vi "Exit.vi"(8 "error in (no error)":errorcluster, 11 "SV_Publisher in":refnum<class "SV_Publisher.lvclass">) -> (0 "error out":errorcluster, 3 "SV_Publisher out":refnum<class "SV_Publisher.lvclass">)   [LabVIEW 2019, in "SV_Publisher.lvclass"]
uses:
  SV_Publisher.lvclass
  Data.ctl
  SV_Publisher.lvclass/SV_Publisher.ctl
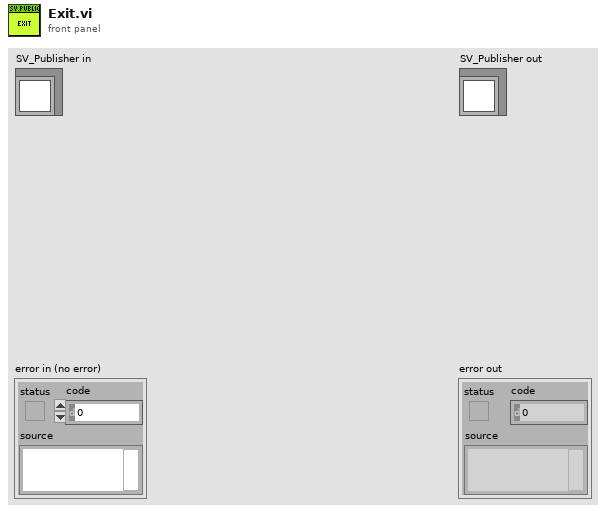
[diagram p1: front panel]
types:
  T1 = typedef "SV_Publisher.lvclass/Data.ctl" = cluster{"Name":string, "Value":variant}
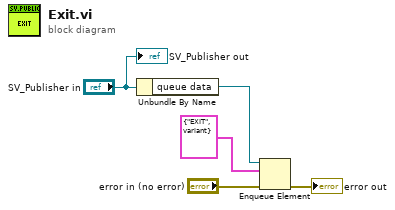
[diagram p0: block diagram]
diagram:
  n1 = Unbundle By Name("SV_Publisher in") -> ("queue data"=w4:refnum<queue>)
  n2 = Enqueue Element(queue=w4, element=T1 {"Name"="EXIT", "Value"=variant}, error in (no error)="error in (no error)") -> (error out=→"error out":errorcluster)  [unwired: 1 in, 2 out]
  "SV_Publisher out" <- "SV_Publisher in"
